vi "XLP80_Datalog_WriteData.vi"(8 "error in":errorcluster caption="error out") -> (0 "error OUT":errorcluster caption="error out")   [LabVIEW 2021]
doc: "Es wird der Dateiname überprüft und die erste Zeile des Files erzeugt (Spaltenbezeichnung). In der ersten Zeile stehen die Kanalnamen und die Zeit, in der zweiten Zeile stehen die Einheiten."
uses:
  XLP80_State_V001.llb/XLP80_State_TDefEnumStateDatalog.ctl
  XLP80_General_Libs/WL_Libs_V14.25/WL_Datalog_V14.00.llb/WL_Datalog_Global.vi
  XLP80_State_V001.llb/XLP80_State_Globals.vi
  XLP80_General_Libs/WL_Libs_V14.25/WL_Profile_V14.00.llb/WL_Profile_Globals.vi
  XLP80_Datalog_Globals.vi
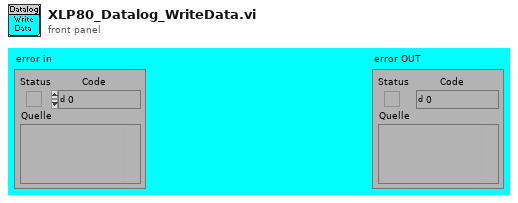
[diagram p1: front panel]
types:
  T1 = typedef "XLP80_State_TDefEnumStateDatalog.ctl" = enum16{"default", "StartLog", "Log", "StopLog", "NewFile"}
  T2 = typedef "WL_Datalog_TypeDefClusterDatalog.ctl" = cluster{"FileName":path, "SaveRate":u32, "but_Save":bool, "but_SnapShot":bool, "Comment":string}
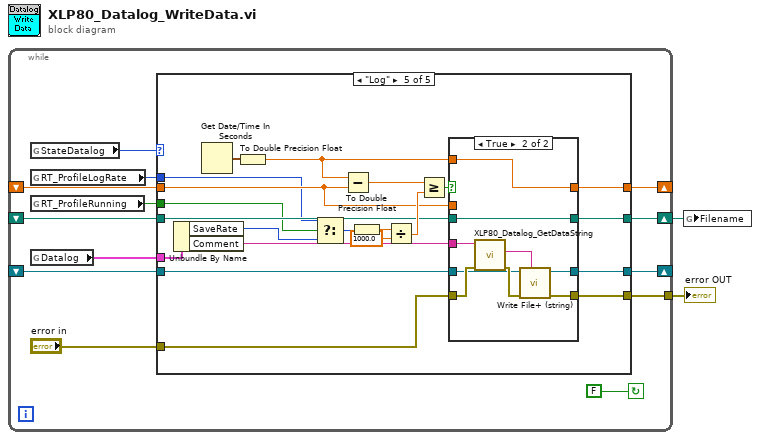
[diagram p0: block diagram]
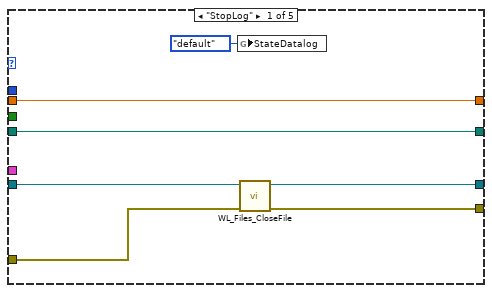
[diagram p2: hidden frame]
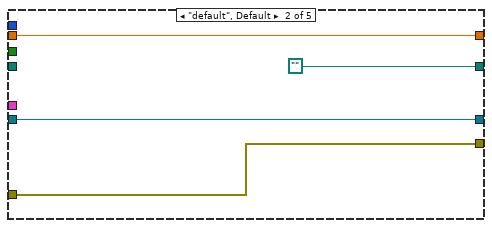
[diagram p3: hidden frame]
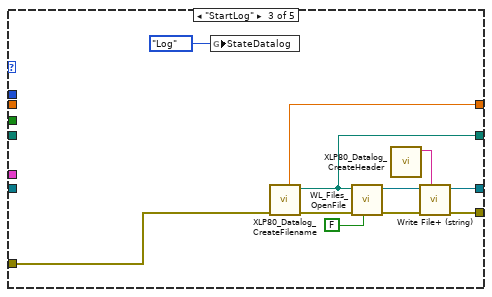
[diagram p4: hidden frame]
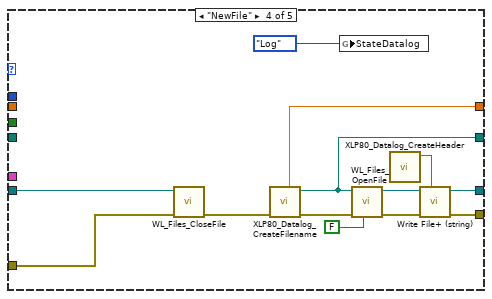
[diagram p5: hidden frame]
diagram:
  n1 = while {
    shift-right: [w14] -> _
    shift-left: _ -> [w13]
    shift-right: [w10] -> w2
    shift-left: _ -> [w9]
    shift-right: [w8] -> _
    shift-left: _ -> [w7]
    tunnel: [w5] -> w1
    stop <- FALSE continue-if-true
    n2 = global read "XLP80_State_Globals.vi" "StateDatalog"() -> (w6:T1)
    n3 = global read "WL_Profile_Globals.vi" "RT_ProfileLogRate"() -> (w3:u32)
    n4 = global read "WL_Profile_Globals.vi" "RT_ProfileRunning"() -> (w4:bool)
    n5 = global read "WL_Datalog_Global.vi" "Datalog"() -> (w11:T2)
    n6 = case shown="\"Log\"" w6 {
      tunnel: [w22 w26 w29 w43 w61] -> w14
      tunnel: w13 -> [w22 w26 _ _ w62]
      tunnel: "error in" -> [w20 w25 w32 w41 w53]
      tunnel: [w19 w25 w35 w48 w58] -> w5
      tunnel: w11 -> [_ _ _ _ w64]
      tunnel: [w21 path "" w30 w44 w60] -> w10
      tunnel: w9 -> [w21 _ _ _ w63]
      tunnel: [w17 w24 w33 w46 w59] -> w8
      tunnel: w7 -> [w18 w24 _ w42 w65]
      tunnel: w4 -> [_ _ _ _ w57]
      tunnel: w3 -> [_ _ _ _ w52]
      frame "StopLog" {
        n7 = global write "XLP80_State_Globals.vi" "StateDatalog"(XLP80_State_TDefEnumStateDatalog."default" ("StateDatalog")) -> ()
        n8 = call "WL_Files_CloseFile.vi"("error in"=w20, "refnum"=w18) -> ("error out"=w19:errorcluster, "refnum"=w17:refnum<file>)  [unwired: 7 in, 1 out]
      }
      frame "default", Default {
      }
      frame "StartLog" {
        n9 = global write "XLP80_State_Globals.vi" "StateDatalog"(XLP80_State_TDefEnumStateDatalog."Log" ("StateDatalog")) -> ()
        n10 = call "XLP80_Datalog_CreateFilename.vi"("error in"=w32) -> ("error out"=w31:errorcluster, "Path"=w30:path, "LogStartTime"=w29:dbl)  [unwired: 8 in]
        n11 = call "WL_Files_OpenFile.vi"("append to file? (new file:F)"=FALSE, "error in"=w31, "file path"=w30) -> ("error out"=w36:errorcluster, "refnum out"=w34:refnum<file>)  [unwired: 6 in, 1 out]
        n12 = call "XLP80_Datalog_CreateHeader.vi"() -> ("Header"=w27:string)  [unwired: 11 in]
        n13 = call <vilib>:"Write File+ (string).vi"("string"=w27, "error in (no error)"=w36, "refnum"=w34) -> ("error out"=w35:errorcluster, "dup refnum"=w33:refnum<file>)  [unwired: 4 in, 1 out]
      }
      frame "NewFile" {
        n14 = call "WL_Files_CloseFile.vi"("error in"=w41, "refnum"=w42) -> ("error out"=w40:errorcluster)  [unwired: 7 in, 2 out]
        n15 = call "XLP80_Datalog_CreateFilename.vi"("error in"=w40) -> ("error out"=w45:errorcluster, "Path"=w44:path, "LogStartTime"=w43:dbl)  [unwired: 8 in]
        n16 = global write "XLP80_State_Globals.vi" "StateDatalog"(XLP80_State_TDefEnumStateDatalog."Log" ("StateDatalog")) -> ()
        n17 = call "WL_Files_OpenFile.vi"("append to file? (new file:F)"=FALSE, "error in"=w45, "file path"=w44) -> ("error out"=w49:errorcluster, "refnum out"=w47:refnum<file>)  [unwired: 6 in, 1 out]
        n18 = call "XLP80_Datalog_CreateHeader.vi"() -> ("Header"=w38:string)  [unwired: 11 in]
        n19 = call <vilib>:"Write File+ (string).vi"("string"=w38, "error in (no error)"=w49, "refnum"=w47) -> ("error out"=w48:errorcluster, "dup refnum"=w46:refnum<file>)  [unwired: 4 in, 1 out]
      }
      frame "Log" {
        n20 = Unbundle By Name(w64) -> ("SaveRate"=w54:u32, "Comment"=w68:string)
        n21 = Get Date/Time In Seconds() -> (seconds since 1Jan1904=w70:timestamp)
        n22 = To Double Precision Float(number=w70) -> (double precision float=w71:dbl)
        n23 = Select(t=w52, s=w57, f=w54) -> (s? t:f=w55:u32)
        n24 = Subtract(x=w71, y=w62) -> (x-y=w66:dbl)
        n25 = To Double Precision Float(number=w55) -> (double precision float=w51:dbl)
        n26 = Divide(x=w51, y=1000.0) -> (x/y=w69:dbl)
        n27 = Greater Or Equal?(x=w66, y=w69) -> (x >= y?=w67:bool)
        n28 = case shown="True" w67 {
          tunnel: [w75 w84] -> w61
          tunnel: w71 -> [_ w84]
          tunnel: w62 -> [w75 _]
          tunnel: w53 -> [w74 w83]
          tunnel: [w74 w79] -> w58
          tunnel: w68 -> [_ w82]
          tunnel: w63 -> [w73 w81]
          tunnel: [w73 w81] -> w60
          tunnel: [w72 w77] -> w59
          tunnel: w65 -> [w72 w76]
          frame False {
          }
          frame True {
            n29 = call "XLP80_Datalog_GetDataString.vi"("error in"=w83, "Comment"=w82) -> ("error OUT"=w80:errorcluster, "String"=w78:string)  [unwired: 8 in]
            n30 = call <vilib>:"Write File+ (string).vi"("string"=w78, "error in (no error)"=w80, "refnum"=w76) -> ("error out"=w79:errorcluster, "dup refnum"=w77:refnum<file>)  [unwired: 4 in, 1 out]
          }
        }
      }
    }
  }
  "error OUT" <- w1
  n31 = global write "XLP80_Datalog_Globals.vi" "Filename"(w2) -> ()
